vi "Cost.vi"(8 "error in (no error)":errorcluster caption="错误输入（无错误）", 11 "Soy 输入":refnum<class "Soy.lvclass">) -> (0 "error out":errorcluster caption="错误输出", 2 "cost":dbl format="%#.3f", 3 "Soy 输出":refnum<class "Soy.lvclass">)   [LabVIEW 2016, in "Soy.lvclass"]
uses:
  Soy.lvclass
  Soy.lvclass/Soy.ctl
  Beverage.lvclass
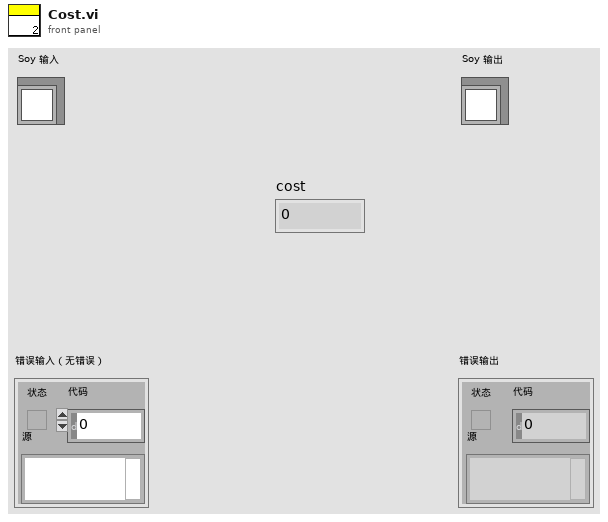
[diagram p1: front panel]
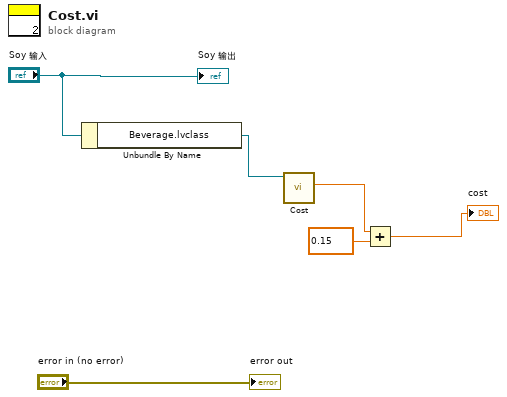
[diagram p0: block diagram]
diagram:
  n1 = Unbundle By Name("Soy 输入") -> ("Beverage.lvclass"=w4:refnum<class "Beverage.lvclass">)
  n2 = call-dynamic "Cost.vi"("Beverage 输入"=w4) -> ("cost"=w3:dbl)  [unwired: 8 in, 2 out]
  n3 = Add(x=w3, y=0.15) -> (x+y=→"cost":dbl)
  "error out" <- "error in (no error)"
  "Soy 输出" <- "Soy 输入"
